vi "Init Hardware.vi"(8 "error in (no error)":errorcluster, 11 "SRS Lockin Driver in":refnum<class "SRS Lockin Driver.lvclass">) -> (0 "error out":errorcluster, 3 "SRS Lockin Driver out":refnum<class "SRS Lockin Driver.lvclass">)   [LabVIEW 2019, in "SRS Lockin Driver.lvclass"]
uses:
  SRS Lockin Driver.lvclass
  C:/GitHub/NHMFL_Core/Libraries/Instruments/Instrument Driver/Instrument Driver.lvclass
  Instrument Driver/Instrument Driver.lvclass/Instrument Driver.ctl
  Instrument Driver/Read Recorder name.vi
  Instrument Driver/Write Channel names.vi
  Instrument Driver/Write Channel units.vi
  Simple VISA Reader/Simple VISA Reader Driver.lvclass
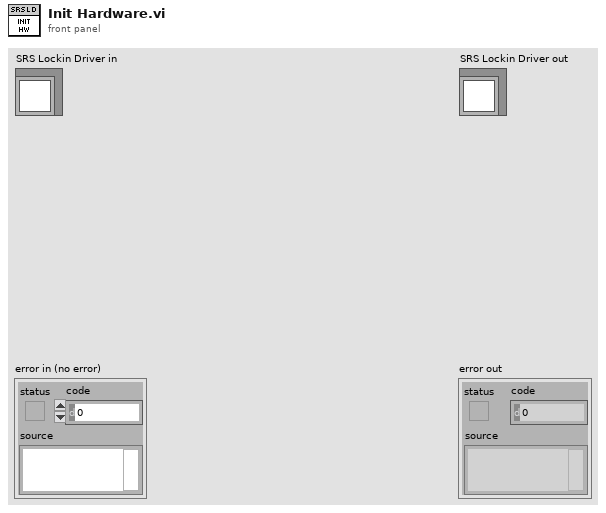
[diagram p1: front panel]
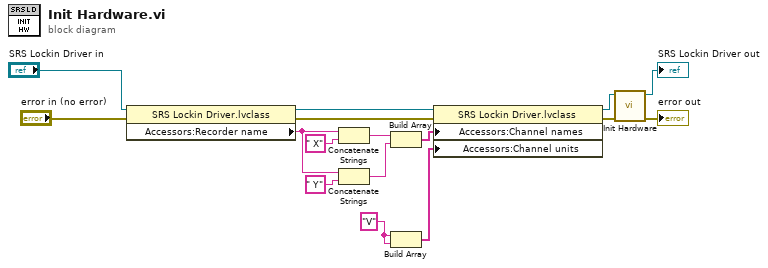
[diagram p0: block diagram]
diagram:
  w1 = "V"
  n1 = property class="SRS Lockin Driver.lvclass"(reference="SRS Lockin Driver in", error in="error in (no error)") -> (reference out=w13:refnum<class "SRS Lockin Driver.lvclass">, error out=w14:errorcluster, "Accessors:Recorder name"=w4:string)
  n2 = Concatenate Strings(w4, " X") -> (w5:string)
  n3 = Concatenate Strings(w4, " Y") -> (w2:string)
  n4 = Build Array(w5, w2) -> (w11:string[])
  n5 = Build Array(w1, w1) -> (w12:string[])
  n6 = property class="SRS Lockin Driver.lvclass"(reference=w13, error in=w14, "Accessors:Channel names"=w11, "Accessors:Channel units"=w12) -> (reference out=w7:refnum<class "SRS Lockin Driver.lvclass">, error out=w8:errorcluster)
  n7 = call-parent "Init Hardware.vi"("error in (no error)"=w8, "Instrument Driver in"=w7) -> ("error out"=→"error out":errorcluster, "Instrument Driver out"=→"SRS Lockin Driver out":refnum<class "SRS Lockin Driver.lvclass">)  [unwired: 8 in]
